vi "Send.vi"(8 "error in":errorcluster, 10 "ICommunicate":refnum<class "ICommunicate.lvclass">, 11 "CANopen Message in":refnum<class "CANopen Message.lvclass">) -> (0 "error out":errorcluster, 3 "CANopen Message out":refnum<class "CANopen Message.lvclass">)   [LabVIEW 2020, in "CANopen.lvlib" / "CANopen Message.lvclass"]
uses:
  CANopen Message.lvclass
  HAL/Source/Interfaces/ICommunicate/ICommunicate.lvclass
  HAL/Source/Interfaces/IMessage/IMessage.lvclass
  HAL/Source/Messages/CAN CC Frame/CAN CC Frame.lvclass
  CANopen Message.lvclass/CANopen Message.ctl
  Logging/Trace Type.ctl
  Logging/CANopen Logging.lvlib
  Logging/Log Level.vi
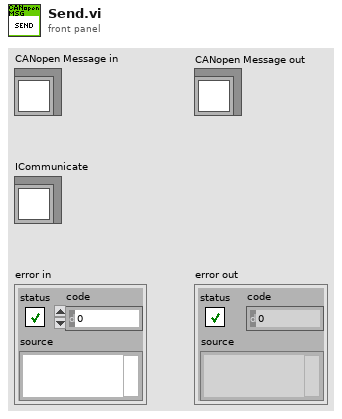
[diagram p1: front panel]
types:
  T1 = enum16{"Error", "Warn", "Info", "Debug", "Trace"}
  T2 = typedef "CANopen Logging.lvlib/Trace Type.ctl" = enum16{"Undefined", "Sent", "Received", "SDO Transfer"}
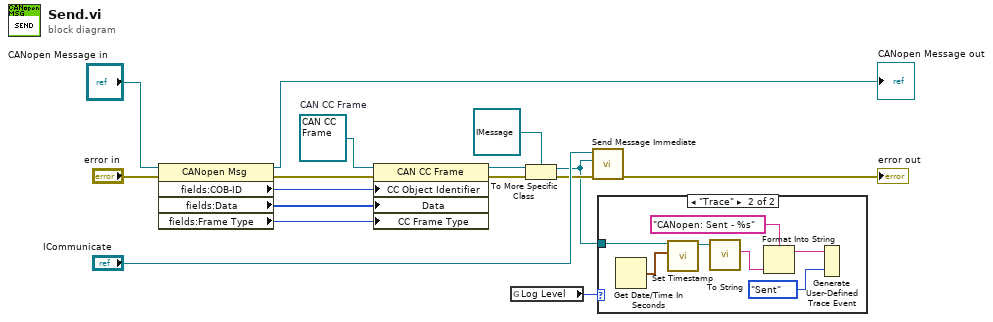
[diagram p0: block diagram]
diagram:
  w4 = refnum<class "CAN CC Frame.lvclass"> refnum  # CAN CC Frame
  n1 = property class="CANopen Msg"(reference="CANopen Message in", error in="error in") -> (reference out=→"CANopen Message out":refnum<class "CANopen Message.lvclass">, error out=w11:errorcluster, "fields:COB-ID"=w10:u32, "fields:Data"=w9:u8[], "fields:Frame Type"=w5:enum8{"Data", "Remote", "Error", "Overload"})
  n2 = property class="CAN CC Frame"(reference=w4, error in=w11, "CC Object Identifier"=w10, "Data"=w9, "CC Frame Type"=w5) -> (reference out=w3:refnum<class "CAN CC Frame.lvclass">, error out=w15:errorcluster)
  n3 = global read "Log Level.vi" "Log Level"() -> (w1:T1)
  n4 = To More Specific Class(target class=refnum<class "IMessage.lvclass"> refnum ("IMessage"), reference=w3, error in=w15) -> (specific class reference=w2:refnum<class "IMessage.lvclass">, error out=w7:errorcluster)
  n5 = call-dynamic "Send Message Immediate.vi"("error in"=w7, "IMessage"=w2, "ICommunicate in"="ICommunicate") -> ("error out"=→"error out":errorcluster)  [unwired: 7 in, 1 out]
  n6 = case shown="\"Trace\"" w1 {
    tunnel: w2 -> [_ w19]
    frame Default {
    }
    frame "Trace" {
      n7 = Get Date/Time In Seconds() -> (seconds since 1Jan1904=w17:timestamp)
      n8 = call-dynamic "Set Timestamp.vi"("Time Stamp"=w17, "IMessage in"=w19) -> ("IMessage out"=w18:refnum<class "IMessage.lvclass">)  [unwired: 8 in, 1 out]
      n9 = call-dynamic "To String.vi"("IMessage in"=w18) -> ("Stringified"=w20:string)  [unwired: 8 in, 2 out]
      n10 = Format Into String(format string="CANopen: Sent - %s", w20) -> (resulting string=w23:string)  [unwired: 2 in, 1 out]
      n11 = Generate User-Defined Trace Event(1:Trace_Type."Sent" ("Trace Type"), 2:w23) -> ()
    }
  }
